vi "operations.vi"(1 "B":dbl, 2 "Operation":string(combo), 3 "A":dbl) -> (0 "Result":dbl)   [LabVIEW 2021]
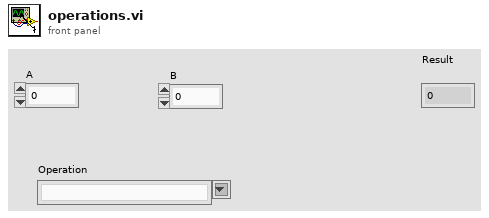
[diagram p1: front panel]
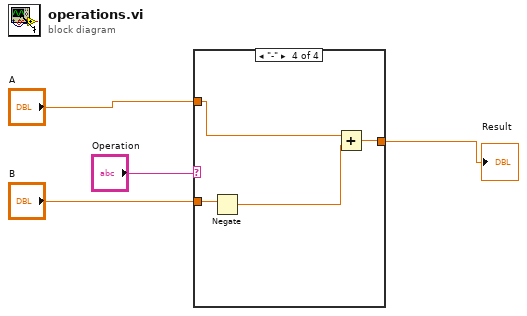
[diagram p0: block diagram]
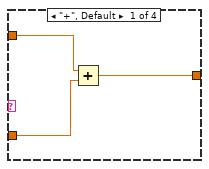
[diagram p2: hidden frame]
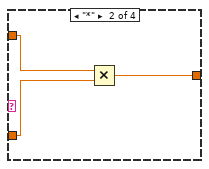
[diagram p3: hidden frame]
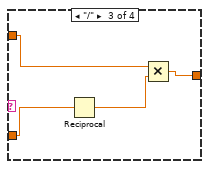
[diagram p4: hidden frame]
diagram:
  n1 = case shown="\"-\"" "Operation" {
    tunnel: "A" -> [w7 w10 w11 w15]
    tunnel: "B" -> [w6 w9 w13 w17]
    tunnel: [w5 w8 w14 w18] -> w1
    frame "+", Default {
      n2 = Add(x=w7, y=w6) -> (x+y=w5:dbl)
    }
    frame "*" {
      n3 = Multiply(x=w10, y=w9) -> (x*y=w8:dbl)
    }
    frame "/" {
      n4 = Reciprocal(x=w13) -> (1/x=w12:dbl)
      n5 = Multiply(x=w11, y=w12) -> (x*y=w14:dbl)
    }
    frame "-" {
      n6 = Negate(x=w17) -> (-x=w16:dbl)
      n7 = Add(x=w15, y=w16) -> (x+y=w18:dbl)
    }
  }
  "Result" <- w1
